vi "gjson_ExtractType.vi"(6 "Encaps Array Info":T1, 8 "error in":errorcluster, 11 "JSON Line":string) -> (0 "error out":errorcluster, 1 "Item Name":cluster{"Hierarchy":string, "Item Name":string}, 2 "Extracted Content":string, 3 "Extracted Type":string, 4 "Encaps Array Info Out":T1)   [LabVIEW 2015, in "Json2Labv.lvlib"]
uses:
  Json2Labv.lvlib
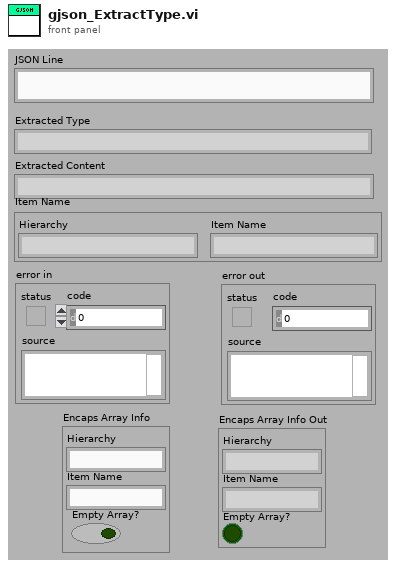
[diagram p1: front panel]
types:
  T1 = cluster{"Hierarchy":string, "Item Name":string, "Empty Array?":bool}
  T2 = cluster{"token string":string, "token string":string}
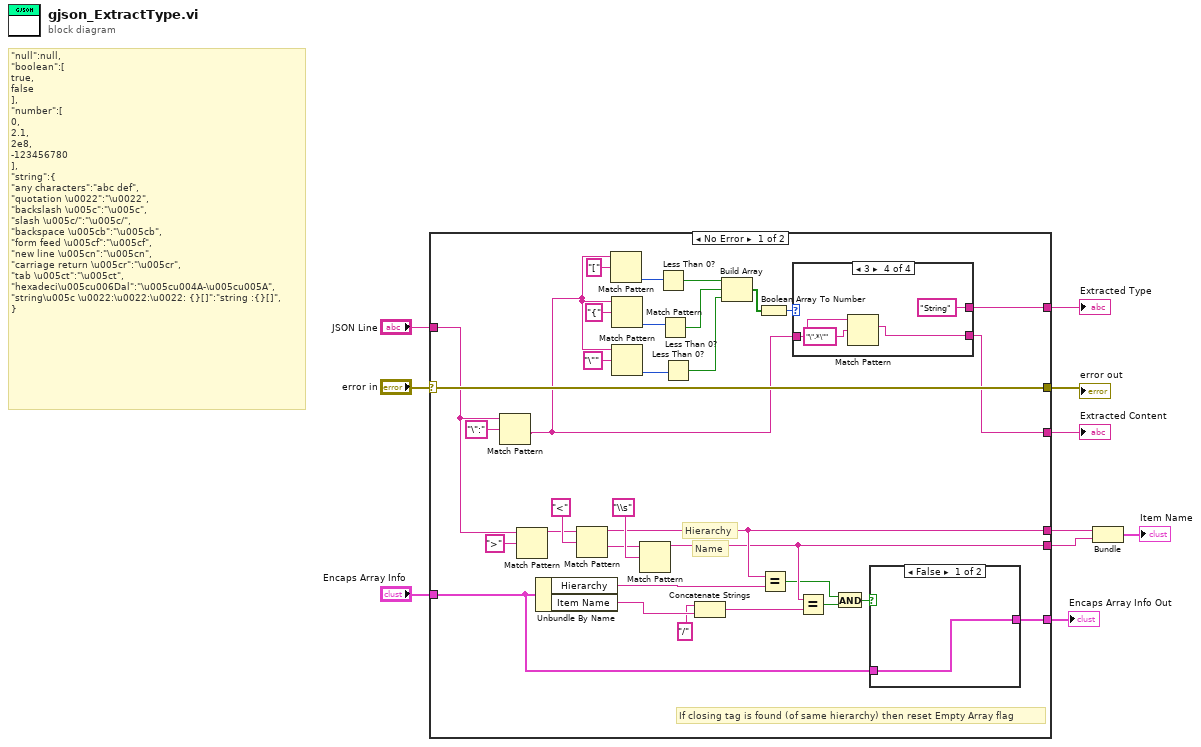
[diagram p0: block diagram]
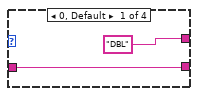
[diagram p2: hidden frame]
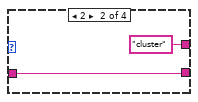
[diagram p3: hidden frame]
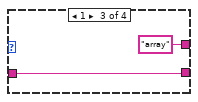
[diagram p4: hidden frame]
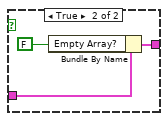
[diagram p5: hidden frame]
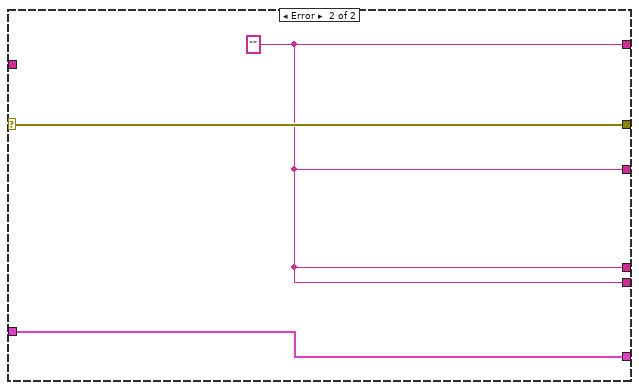
[diagram p6: hidden frame]
diagram:
  # "\"null\":null,\n\"boolean\":[\ntrue,\nfalse\n],\n\"number\":[\n0,\n2.1,\n2e8,\n-123456780\n],\n\"string\":{\n\"any characters\":\"abc def\",\n\"quotation \\u0022\":\"\\u0022\",\n\"backslash \\u005c\":\"\\u005c\",\n\"slash \\u005c/\":\"\\u005c/\",\n\"backspace \\u005cb\":\"\\u005cb\",\n\"form feed \\u005cf\":\"\\u005cf\",\n\"new line \\u005cn\":\"\\u005cn\",\n\"carriage return \\u005cr\":\"\\u005cr\",\n\"tab \\u005ct\":\"\\u005ct\",\n\"hexadeci\\u005cu006Dal\":\"\\u005cu004A-\\u005cu005A\",\n\"string\\u005c \\u0022:\\u0022:\\u0022: {}[]\":\"string :{}[]\",\n}"
  n1 = case shown="No Error" "error in" {
    selector: "error in" -> [w26 w60]
    tunnel: [w18 w59] -> w10
    tunnel: "JSON Line" -> [w16 _]
    tunnel: [w26 w60] -> w8
    tunnel: [w11 w59] -> w6
    tunnel: [w38 w59] -> w5
    tunnel: [w33 w59] -> w4
    tunnel: "Encaps Array Info" -> [w29 w58]
    tunnel: [w28 w58] -> w1
    frame No Error {
      # "If closing tag is found (of same hierarchy) then reset Empty Array flag"
      # "Name"
      # "Hierarchy"
      n2 = Match Pattern(string=w16, regular expression="\":") -> (after substring=w12:string)  [unwired: 1 in, 3 out]
      n3 = Match Pattern(string=w16, regular expression=">") -> (before substring=w40:string)  [unwired: 1 in, 3 out]
      n4 = Unbundle By Name(w29) -> ("Hierarchy"=w37:string, "Item Name"=w36:string)
      n5 = Match Pattern(string=w40, regular expression="<") -> (before substring=w38:string, after substring=w42:string)  [unwired: 1 in, 2 out]
      n6 = Match Pattern(string=w12, regular expression="[") -> (offset past match=w23:i32)  [unwired: 1 in, 3 out]
      n7 = Match Pattern(string=w12, regular expression="{") -> (offset past match=w25:i32)  [unwired: 1 in, 3 out]
      n8 = Match Pattern(string=w12, regular expression="\"") -> (offset past match=w14:i32)  [unwired: 1 in, 3 out]
      n9 = Match Pattern(string=w42, regular expression="\\s") -> (before substring=w33:string)  [unwired: 1 in, 3 out]
      n10 = Less Than 0?(x=w23) -> (x < 0?=w22:bool)
      n11 = Less Than 0?(x=w25) -> (x < 0?=w21:bool)
      n12 = Less Than 0?(x=w14) -> (x < 0?=w13:bool)
      n13 = Concatenate Strings("/" ("string"), w36) -> (w34:string)
      n14 = Build Array(w22, w21, w13) -> (w20:bool[])
      n15 = Boolean Array To Number(Boolean array=w20) -> (number=w19:u32)
      n16 = Equal?(x=w38, y=w37) -> (x = y?=w31:bool)
      n17 = case shown="3" w19 {
        tunnel: ["DBL" "cluster" "array" "String"] -> w18
        tunnel: w12 -> [w44 w46 w48 w52]
        tunnel: [w44 w46 w48 w51] -> w11
        frame 0, Default {
        }
        frame 2 {
        }
        frame 1 {
        }
        frame 3 {
          n18 = Match Pattern(string=w52, regular expression="\".*\"") -> (match substring=w51:string)  [unwired: 1 in, 3 out]
        }
      }
      n19 = Equal?(x=w33, y=w34) -> (x = y?=w32:bool)
      n20 = And(x=w31, y=w32) -> (x .and. y?=w30:bool)
      n21 = case shown="False" w30 {
        tunnel: w29 -> [w54 w57]
        tunnel: [w54 w55] -> w28
        frame False {
        }
        frame True {
          n22 = Bundle By Name(cluster=w57, "Empty Array?"=FALSE) -> (w55:T1)
        }
      }
    }
    frame Error {
      w59 = "" ("token string")
    }
  }
  "Extracted Type" <- w10
  "error out" <- w8
  "Extracted Content" <- w6
  "Encaps Array Info Out" <- w1
  n23 = Bundle("token string"=w5, "token string"=w4) -> (→"Item Name":T2)  [unwired: 1 in]
